vi "nanocal -- nuclear schottky fit V8.vi"() -> ()   [LabVIEW 2021] (continued)
0.011257222829   ,  \"σηlogτN\" -> 0.184131010310   ,  \"σlogτ1\" -> 0.004582504926   ,  \"σlogτS\" -> 0.002840955825   ,  \"σlogτN\" -> 0.002523601752   ,  \"σητ1\" -> 0.013755317417   ,  \"σητS \" -> 0.001255629993   ,  \"σητN\" -> 0.084667169226    |>   , \r\"IDS0627_220611_RAW_cal__sam_\" ->   <|    \"ζ\" -> 0.000000000000   ,  \"τ1\" -> 0.000000000000   ,  \"τS\" -> 0.000000000000   ,  \"τN\" -> 0.000000000000   ,  \"τC\" -> 0.000000000000   ,  \"κ0\" -> 0.000000000000   ,  \"mm1\" -> 0.000000000000   ,  \"mm2\" -> 0.000000000000   ,  \"mm3\" -> 0.000000000000   ,  \"T\" -> 0.120000000000   ,  \"B\" -> 10.000000000000   ,  \"θ\" -> 90.000000000000   ,  \"Reoff\" -> 0.000000000000   ,  \"Imoff\" -> 0.000000000000   ,  \"στ1\" -> 0.000000000000   ,  \"στS\" -> 0.000000000000   ,  \"στN\" -> 0.000000000000   ,  \"τ11 \" -> 0.000000000000   ,  \"τ12\" -> 0.000000000000   ,  \"τ22\" -> 0.000000000000   ,  \"τN1\" -> 0.000000000000   ,  \"τN2\" -> 0.000000000000   ,  \"σηlogτ1 \" -> 0.000000000000   ,  \"σηlogτS\" -> 0.000000000000   ,  \"σηlogτN\" -> 0.000000000000   ,  \"σlogτ1\" -> 0.000000000000   ,  \"σlogτS\" -> 0.000000000000   ,  \"σlogτN\" -> 0.000000000000   ,  \"σητ1\" -> 0.000000000000   ,  \"σητS \" -> 0.000000000000   ,  \"σητN\" -> 0.000000000000    |>   , \r\"IDS0628_220611_RAW_cal__ref_\" ->   <|    \"ζ\" -> 0.152770220737   ,  \"τ1\" -> 0.036198364925   ,  \"τS\" -> 0.033549808091   ,  \"τN\" -> 0.027206802922   ,  \"τC\" -> 0.001036197063   ,  \"κ0\" -> 0.000000001265   ,  \"mm1\" -> 0.000134182447   ,  \"mm2\" -> 0.015662270095   ,  \"mm3\" -> 0.091476521334   ,  \"T\" -> 0.250000000000   ,  \"B\" -> 10.000000000000   ,  \"θ\" -> 90.000000000000   ,  \"Reoff\" -> 0.000000000000   ,  \"Imoff\" -> 0.000000000000   ,  \"στ1\" -> 0.000013390131   ,  \"στS\" -> 0.000002421606   ,  \"στN\" -> 0.000006177026   ,  \"τ11 \" -> 0.000000000000   ,  \"τ12\" -> 0.000000000000   ,  \"τ22\" -> 0.000000000000   ,  \"τN1\" -> 0.000000000000   ,  \"τN2\" -> 0.000000000000   ,  \"σηlogτ1 \" -> 0.116147333813   ,  \"σηlogτS\" -> 0.002721053400   ,  \"σηlogτN\" -> 0.134955883548   ,  \"σlogτ1\" -> 0.000369909834   ,  \"σlogτS\" -> 0.000072179437   ,  \"σlogτN\" -> 0.000227039759   ,  \"σητ1\" -> 0.004204343574   ,  \"σητS \" -> 0.000091290819   ,  \"σητN\" -> 0.003671718127    |>   , \r\"IDS0628_220611_RAW_cal__sam_\" ->   <|    \"ζ\" -> 0.000000000000   ,  \"τ1\" -> 0.000000000000   ,  \"τS\" -> 0.000000000000   ,  \"τN\" -> 0.000000000000   ,  \"τC\" -> 0.000000000000   ,  \"κ0\" -> 0.000000000000   ,  \"mm1\" -> 0.000000000000   ,  \"mm2\" -> 0.000000000000   ,  \"mm3\" -> 0.000000000000   ,  \"T\" -> 0.250000000000   ,  \"B\" -> 10.000000000000   ,  \"θ\" -> 90.000000000000   ,  \"Reoff\" -> 0.000000000000   ,  \"Imoff\" -> 0.000000000000   ,  \"στ1\" -> 0.000000000000   ,  \"στS\" -> 0.000000000000   ,  \"στN\" -> 0.000000000000   ,  \"τ11 \" -> 0.000000000000   ,  \"τ12\" -> 0.000000000000   ,  \"τ22\" -> 0.000000000000   ,  \"τN1\" -> 0.000000000000   ,  \"τN2\" -> 0.000000000000   ,  \"σηlogτ1 \" -> 0.000000000000   ,  \"σηlogτS\" -> 0.000000000000   ,  \"σηlogτN\" -> 0.000000000000   ,  \"σlogτ1\" -> 0.000000000000   ,  \"σlogτS\" -> 0.000000000000   ,  \"σlogτN\" -> 0.000000000000   ,  \"σητ1\" -> 0.000000000000   ,  \"σητS \" -> 0.000000000000   ,  \"σητN\" -> 0.000000000000    |>   , \r\"IDS0629_220611_RAW_cal__ref_\" ->   <|    \"ζ\" -> 0.104961058193   ,  \"τ1\" -> 0.030489437824   ,  \"τS\" -> 0.030011872176   ,  \"τN\" -> 0.014021025099   ,  \"τC\" -> 0.001158647608   ,  \"κ0\" -> 0.000000001606   ,  \"mm1\" -> 0.000106671353   ,  \"mm2\" -> 0.016335963882   ,  \"mm3\" -> 0.063860086965   ,  \"T\" -> 0.300000000000   ,  \"B\" -> 10.000000000000   ,  \"θ\" -> 90.000000000000   ,  \"Reoff\" -> 0.000000000000   ,  \"Imoff\" -> 0.000000000000   ,  \"στ1\" -> 0.000007085631   ,  \"στS\" -> 0.000000880275   ,  \"στN\" -> 0.000001925171   ,  \"τ11 \" -> 0.000000000000   ,  \"τ12\" -> 0.000000000000   ,  \"τ22\" -> 0.000000000000   ,  \"τN1\" -> 0.000000000000   ,  \"τN2\" -> 0.000000000000   ,  \"σηlogτ1 \" -> 0.117123612292   ,  \"σηlogτS\" -> 0.001807335056   ,  \"σηlogτN\" -> 0.132991316128   ,  \"σlogτ1\" -> 0.000232396245   ,  \"σlogτS\" -> 0.000029330901   ,  \"σlogτN\" -> 0.000137306042   ,  \"σητ1\" -> 0.003571033095   ,  \"σητS \" -> 0.000054241509   ,  \"σητN\" -> 0.001864674581    |>   , \r\"IDS0629_220611_RAW_cal__sam_\" ->   <|    \"ζ\" -> 0.000000000000   ,  \"τ1\" -> 0.000000000000   ,  \"τS\" -> 0.000000000000   ,  \"τN\" -> 0.000000000000   ,  \"τC\" -> 0.000000000000   ,  \"κ0\" -> 0.000000000000   ,  \"mm1\" -> 0.000000000000   ,  \"mm2\" -> 0.000000000000   ,  \"mm3\" -> 0.000000000000   ,  \"T\" -> 0.300000000000   ,  \"B\" -> 10.000000000000   ,  \"θ\" -> 90.000000000000   ,  \"Reoff\" -> 0.000000000000   ,  \"Imoff\" -> 0.000000000000   ,  \"στ1\" -> 0.000000000000   ,  \"στS\" -> 0.000000000000   ,  \"στN\" -> 0.000000000000   ,  \"τ11 \" -> 0.000000000000   ,  \"τ12\" -> 0.000000000000   ,  \"τ22\" -> 0.000000000000   ,  \"τN1\" -> 0.000000000000   ,  \"τN2\" -> 0.000000000000   ,  \"σηlogτ1 \" -> 0.000000000000   ,  \"σηlogτS\" -> 0.000000000000   ,  \"σηlogτN\" -> 0.000000000000   ,  \"σlogτ1\" -> 0.000000000000   ,  \"σlogτS\" -> 0.000000000000   ,  \"σlogτN\" -> 0.000000000000   ,  \"σητ1\" -> 0.000000000000   ,  \"σητS \" -> 0.000000000000   ,  \"σητN\" -> 0.000000000000    |>   , \r\"IDS0630_220611_RAW_cal__ref_\" ->   <|    \"ζ\" -> 0.075687079530   ,  \"τ1\" -> 0.025692917456   ,  \"τS\" -> 0.027518005635   ,  \"τN\" -> 0.007256477389   ,  \"τC\" -> 0.001413406836   ,  \"κ0\" -> 0.000000002017   ,  \"mm1\" -> 0.000095205662   ,  \"mm2\" -> 0.016621150094   ,  \"mm3\" -> 0.047796430622   ,  \"T\" -> 0.360000000000   ,  \"B\" -> 10.000000000000   ,  \"θ\" -> 90.000000000000   ,  \"Reoff\" -> 0.000000000000   ,  \"Imoff\" -> 0.000000000000   ,  \"στ1\" -> 0.000009211361   ,  \"στS\" -> 0.000000780336   ,  \"στN\" -> 0.000001470575   ,  \"τ11 \" -> 0.000000000000   ,  \"τ12\" -> 0.000000000000   ,  \"τ22\" -> 0.000000000000   ,  \"τN1\" -> 0.000000000000   ,  \"τN2\" -> 0.000000000000   ,  \"σηlogτ1 \" -> 0.121353390675   ,  \"σηlogτS\" -> 0.001216073528   ,  \"σηlogτN\" -> 0.132703139128   ,  \"σlogτ1\" -> 0.000358517508   ,  \"σlogτS\" -> 0.000028357288   ,  \"σlogτN\" -> 0.000202656857   ,  \"σητ1\" -> 0.003117922650   ,  \"σητS \" -> 0.000033463918   ,  \"σητN\" -> 0.000962957328    |>   , \r\"IDS0630_220611_RAW_cal__sam_\" ->   <|    \"ζ\" -> 0.000000000000   ,  \"τ1\" -> 0.000000000000   ,  \"τS\" -> 0.000000000000   ,  \"τN\" -> 0.000000000000   ,  \"τC\" -> 0.000000000000   ,  \"κ0\" -> 0.000000000000   ,  \"mm1\" -> 0.000000000000   ,  \"mm2\" -> 0.000000000000   ,  \"mm3\" -> 0.000000000000   ,  \"T\" -> 0.360000000000   ,  \"B\" -> 10.000000000000   ,  \"θ\" -> 90.000000000000   ,  \"Reoff\" -> 0.000000000000   ,  \"Imoff\" -> 0.000000000000   ,  \"στ1\" -> 0.000000000000   ,  \"στS\" -> 0.000000000000   ,  \"στN\" -> 0.000000000000   ,  \"τ11 \" -> 0.000000000000   ,  \"τ12\" -> 0.000000000000   ,  \"τ22\" -> 0.000000000000   ,  \"τN1\" -> 0.000000000000   ,  \"τN2\" -> 0.000000000000   ,  \"σηlogτ1 \" -> 0.000000000000   ,  \"σηlogτS\" -> 0.000000000000   ,  \"σηlogτN\" -> 0.000000000000   ,  \"σlogτ1\" -> 0.000000000000   ,  \"σlogτS\" -> 0.000000000000   ,  \"σlogτN\" -> 0.000000000000   ,  \"σητ1\" -> 0.000000000000   ,  \"σητS \" -> 0.000000000000   ,  \"σητN\" -> 0.000000000000    |>   , \r\"IDS0631_220611_RAW_cal__ref_\" ->   <|    \"ζ\" -> 0.058935240336   ,  \"τ1\" -> 0.021193518217   ,  \"τS\" -> 0.025799898485   ,  \"τN\" -> 0.004769009758   ,  \"τC\" -> 0.001612077295   ,  \"κ0\" -> 0.000000002413   ,  \"mm1\" -> 0.000084967559   ,  \"mm2\" -> 0.015406650385   ,  \"mm3\" -> 0.039684471765   ,  \"T\" -> 0.420000000000   ,  \"B\" -> 10.000000000000   ,  \"θ\" -> 90.000000000000   ,  \"Reoff\" -> 0.000000000000   ,  \"Imoff\" -> 0.000000000000   ,  \"στ1\" -> 0.000010740234   ,  \"στS\" -> 0.000000797297   ,  \"στN\" -> 0.000001307044   ,  \"τ11 \" -> 0.000000000000   ,  \"τ12\" -> 0.000000000000   ,  \"τ22\" -> 0.000000000000   ,  \"τN1\" -> 0.000000000000   ,  \"τN2\" -> 0.000000000000   ,  \"σηlogτ1 \" -> 0.129682628231   ,  \"σηlogτS\" -> 0.001061043633   ,  \"σηlogτN\" -> 0.134054055610   ,  \"σlogτ1\" -> 0.000506769772   ,  \"σlogτS\" -> 0.000030903120   ,  \"σlogτN\" -> 0.000274070212   ,  \"σητ1\" -> 0.002748431144   ,  \"σητS \" -> 0.000027374818   ,  \"σητN\" -> 0.000639305099    |>   , \r\"IDS0631_220611_RAW_cal__sam_\" ->   <|    \"ζ\" -> 0.000000000000   ,  \"τ1\" -> 0.000000000000   ,  \"τS\" -> 0.000000000000   ,  \"τN\" -> 0.000000000000   ,  \"τC\" -> 0.000000000000   ,  \"κ0\" -> 0.000000000000   ,  \"mm1\" -> 0.000000000000   ,  \"mm2\" -> 0.000000000000   ,  \"mm3\" -> 0.000000000000   ,  \"T\" -> 0.420000000000   ,  \"B\" -> 10.000000000000   ,  \"θ\" -> 90.000000000000   ,  \"Reoff\" -> 0.000000000000   ,  \"Imoff\" -> 0.000000000000   ,  \"στ1\" -> 0.000000000000   ,  \"στS\" -> 0.000000000000   ,  \"στN\" -> 0.000000000000   ,  \"τ11 \" -> 0.000000000000   ,  \"τ12\" -> 0.000000000000   ,  \"τ22\" -> 0.000000000000   ,  \"τN1\" -> 0.000000000000   ,  \"τN2\" -> 0.000000000000   ,  \"σηlogτ1 \" -> 0.000000000000   ,  \"σηlogτS\" -> 0.000000000000   ,  \"σηlogτN\" -> 0.000000000000   ,  \"σlogτ1\" -> 0.000000000000   ,  \"σlogτS\" -> 0.000000000000   ,  \"σlogτN\" -> 0.000000000000   ,  \"σητ1\" -> 0.000000000000   ,  \"σητS \" -> 0.000000000000   ,  \"σητN\" -> 0.000000000000    |>   , \r\"IDS0632_220611_RAW_cal__ref_\" ->   <|    \"ζ\" -> 0.044055217720   ,  \"τ1\" -> 0.018398673141   ,  \"τS\" -> 0.024296902753   ,  \"τN\" -> 0.002237219247   ,  \"τC\" -> 0.001705422897   ,  \"κ0\" -> 0.000000003103   ,  \"mm1\" -> 0.000067596634   ,  \"mm2\" -> 0.015331750366   ,  \"mm3\" -> 0.032407837560   ,  \"T\" -> 0.520000000000   ,  \"B\" -> 10.000000000000   ,  \"θ\" -> 90.000000000000   ,  \"Reoff\" -> 0.000000000000   ,  \"Imoff\" -> 0.000000000000   ,  \"στ1\" -> 0.000025900073   ,  \"στS\" -> 0.000001114973   ,  \"στN\" -> 0.000001649689   ,  \"τ11 \" -> 0.000000000000   ,  \"τ12\" -> 0.000000000000   ,  \"τ22\" -> 0.000000000000   ,  \"τN1\" -> 0.000000000000   ,  \"τN2\" -> 0.000000000000   ,  \"σηlogτ1 \" -> 0.135453082912   ,  \"σηlogτS\" -> 0.000614451179   ,  \"σηlogτN\" -> 0.134477904132   ,  \"σlogτ1\" -> 0.001407714152   ,  \"σlogτS\" -> 0.000045889504   ,  \"σlogτN\" -> 0.000737383723   ,  \"σητ1\" -> 0.002492156998   ,  \"σητS \" -> 0.000014929261   ,  \"σητN\" -> 0.000300856555    |>   , \r\"IDS0632_220611_RAW_cal__sam_\" ->   <|    \"ζ\" -> 0.000000000000   ,  \"τ1\" -> 0.000000000000   ,  \"τS\" -> 0.000000000000   ,  \"τN\" -> 0.000000000000   ,  \"τC\" -> 0.000000000000   ,  \"κ0\" -> 0.000000000000   ,  \"mm1\" -> 0.000000000000   ,  \"mm2\" -> 0.000000000000   ,  \"mm3\" -> 0.000000000000   ,  \"T\" -> 0.520000000000   ,  \"B\" -> 10.000000000000   ,  \"θ\" -> 90.000000000000   ,  \"Reoff\" -> 0.000000000000   ,  \"Imoff\" -> 0.000000000000   ,  \"στ1\" -> 0.000000000000   ,  \"στS\" -> 0.000000000000   ,  \"στN\" -> 0.000000000000   ,  \"τ11 \" -> 0.000000000000   ,  \"τ12\" -> 0.000000000000   ,  \"τ22\" -> 0.000000000000   ,  \"τN1\" -> 0.000000000000   ,  \"τN2\" -> 0.000000000000   ,  \"σηlogτ1 \" -> 0.000000000000   ,  \"σηlogτS\" -> 0.000000000000   ,  \"σηlogτN\" -> 0.000000000000   ,  \"σlogτ1\" -> 0.000000000000   ,  \"σlogτS\" -> 0.000000000000   ,  \"σlogτN\" -> 0.000000000000   ,  \"σητ1\" -> 0.000000000000   ,  \"σητS \" -> 0.000000000000   ,  \"σητN\" -> 0.000000000000    |>   , \r\"IDS0633_220611_RAW_cal__ref_\" ->   <|    \"ζ\" -> 0.034142201059   ,  \"τ1\" -> 0.016889163361   ,  \"τS\" -> 0.022852529077   ,  \"τN\" -> 0.001326577994   ,  \"τC\" -> 0.002278925943   ,  \"κ0\" -> 0.000000003798   ,  \"mm1\" -> 0.000068802803   ,  \"mm2\" -> 0.014993961538   ,  \"mm3\" -> 0.029109959968   ,  \"T\" -> 0.620000000000   ,  \"B\" -> 10.000000000000   ,  \"θ\" -> 90.000000000000   ,  \"Reoff\" -> 0.000000000000   ,  \"Imoff\" -> 0.000000000000   ,  \"στ1\" -> 0.000028192933   ,  \"στS\" -> 0.000000811322   ,  \"στN\" -> 0.000001142735   ,  \"τ11 \" -> 0.000000000000   ,  \"τ12\" -> 0.000000000000   ,  \"τ22\" -> 0.000000000000   ,  \"τN1\" -> 0.000000000000   ,  \"τN2\" -> 0.000000000000   ,  \"σηlogτ1 \" -> 0.138852812126   ,  \"σηlogτS\" -> 0.000419923481   ,  \"σηlogτN\" -> 0.134804184987   ,  \"σlogτ1\" -> 0.001669291277   ,  \"σlogτS\" -> 0.000035502510   ,  \"σlogτN\" -> 0.000861415426   ,  \"σητ1\" -> 0.002345107827   ,  \"σητS \" -> 0.000009596314   ,  \"σητN\" -> 0.000178828265    |>   , \r\"IDS0633_220611_RAW_cal__sam_\" ->   <|    \"ζ\" -> 0.000000000000   ,  \"τ1\" -> 0.000000000000   ,  \"τS\" -> 0.000000000000   ,  \"τN\" -> 0.000000000000   ,  \"τC\" -> 0.000000000000   ,  \"κ0\" -> 0.000000000000   ,  \"mm1\" -> 0.000000000000   ,  \"mm2\" -> 0.000000000000   ,  \"mm3\" -> 0.000000000000   ,  \"T\" -> 0.620000000000   ,  \"B\" -> 10.000000000000   ,  \"θ\" -> 90.000000000000   ,  \"Reoff\" -> 0.000000000000   ,  \"Imoff\" -> 0.000000000000   ,  \"στ1\" -> 0.000000000000   ,  \"στS\" -> 0.000000000000   ,  \"στN\" -> 0.000000000000   ,  \"τ11 \" -> 0.000000000000   ,  \"τ12\" -> 0.000000000000   ,  \"τ22\" -> 0.000000000000   ,  \"τN1\" -> 0.000000000000   ,  \"τN2\" -> 0.000000000000   ,  \"σηlogτ1 \" -> 0.000000000000   ,  \"σηlogτS\" -> 0.000000000000   ,  \"σηlogτN\" -> 0.000000000000   ,  \"σlogτ1\" -> 0.000000000000   ,  \"σlogτS\" -> 0.000000000000   ,  \"σlogτN\" -> 0.000000000000   ,  \"σητ1\" -> 0.000000000000   ,  \"σητS \" -> 0.000000000000   ,  \"σητN\" -> 0.000000000000    |>   , \r\"IDS0634_220612_RAW_cal__ref_\" ->   <|    \"ζ\" -> 0.026094794498   ,  \"τ1\" -> 0.017613964803   ,  \"τS\" -> 0.020608194694   ,  \"τN\" -> 0.000565779347   ,  \"τC\" -> 0.002821541401   ,  \"κ0\" -> 0.000000005177   ,  \"mm1\" -> 0.000063475218   ,  \"mm2\" -> 0.016356491351   ,  \"mm3\" -> 0.025742044177   ,  \"T\" -> 0.820000000000   ,  \"B\" -> 10.000000000000   ,  \"θ\" -> 90.000000000000   ,  \"Reoff\" -> 0.000000000000   ,  \"Imoff\" -> 0.000000000000   ,  \"στ1\" -> 0.000096609701   ,  \"στS\" -> 0.000001077026   ,  \"στN\" -> 0.000001637448   ,  \"τ11 \" -> 0.000000000000   ,  \"τ12\" -> 0.000000000000   ,  \"τ22\" -> 0.000000000000   ,  \"τN1\" -> 0.000000000000   ,  \"τN2\" -> 0.000000000000   ,  \"σηlogτ1 \" -> 0.129941381525   ,  \"σηlogτS\" -> 0.000167044779   ,  \"σηlogτN\" -> 0.132803601967   ,  \"σlogτ1\" -> 0.005484835568   ,  \"σlogτS\" -> 0.000052262034   ,  \"σlogτN\" -> 0.002894146508   ,  \"σητ1\" -> 0.002288782921   ,  \"σητS \" -> 0.000003442491   ,  \"σητN\" -> 0.000075137535    |>   , \r\"IDS0634_220612_RAW_cal__sam_\" ->   <|    \"ζ\" -> 0.000000000000   ,  \"τ1\" -> 0.000000000000   ,  \"τS\" -> 0.000000000000   ,  \"τN\" -> 0.000000000000   ,  \"τC\" -> 0.000000000000   ,  \"κ0\" -> 0.000000000000   ,  \"mm1\" -> 0.000000000000   ,  \"mm2\" -> 0.000000000000   ,  \"mm3\" -> 0.000000000000   ,  \"T\" -> 0.820000000000   ,  \"B\" -> 10.000000000000   ,  \"θ\" -> 90.000000000000   ,  \"Reoff\" -> 0.000000000000   ,  \"Imoff\" -> 0.000000000000   ,  \"στ1\" -> 0.000000000000   ,  \"στS\" -> 0.000000000000   ,  \"στN\" -> 0.000000000000   ,  \"τ11 \" -> 0.000000000000   ,  \"τ12\" -> 0.000000000000   ,  \"τ22\" -> 0.000000000000   ,  \"τN1\" -> 0.000000000000   ,  \"τN2\" -> 0.000000000000   ,  \"σηlogτ1 \" -> 0.000000000000   ,  \"σηlogτS\" -> 0.000000000000   ,  \"σηlogτN\" -> 0.000000000000   ,  \"σlogτ1\" -> 0.000000000000   ,  \"σlogτS\" -> 0.000000000000   ,  \"σlogτN\" -> 0.000000000000   ,  \"σητ1\" -> 0.000000000000   ,  \"σητS \" -> 0.000000000000   ,  \"σητN\" -> 0.000000000000    |>   , \r\"IDS0635_220612_RAW_cal__ref_\" ->   <|    \"ζ\" -> 0.022302849506   ,  \"τ1\" -> 0.019271147098   ,  \"τS\" -> 0.018127459113   ,  \"τN\" -> 0.000191566174   ,  \"τC\" -> 0.003097458701   ,  \"κ0\" -> 0.000000007267   ,  \"mm1\" -> 0.000058053364   ,  \"mm2\" -> 0.018210505050   ,  \"mm3\" -> 0.022827639136   ,  \"T\" -> 1.120000000000   ,  \"B\" -> 10.000000000000   ,  \"θ\" -> 90.000000000000   ,  \"Reoff\" -> 0.000000000000   ,  \"Imoff\" -> 0.000000000000   ,  \"στ1\" -> 0.000470741477   ,  \"στS\" -> 0.000001456602   ,  \"στN\" -> 0.000002601409   ,  \"τ11 \" -> 0.000000000000   ,  \"τ12\" -> 0.000000000000   ,  \"τ22\" -> 0.000000000000   ,  \"τN1\" -> 0.000000000000   ,  \"τN2\" -> 0.000000000000   ,  \"σηlogτ1 \" -> 0.117167586135   ,  \"σηlogτS\" -> 0.000047458198   ,  \"σηlogτN\" -> 0.130090926522   ,  \"σlogτ1\" -> 0.024427268103   ,  \"σlogτS\" -> 0.000080353339   ,  \"σlogτN\" -> 0.013579690528   ,  \"σητ1\" -> 0.002257953787   ,  \"σητS \" -> 0.000000860297   ,  \"σητN\" -> 0.000024921021    |>   , \r\"IDS0635_220612_RAW_cal__sam_\" ->   <|    \"ζ\" -> 0.000000000000   ,  \"τ1\" -> 0.000000000000   ,  \"τS\" -> 0.000000000000   ,  \"τN\" -> 0.000000000000   ,  \"τC\" -> 0.000000000000   ,  \"κ0\" -> 0.000000000000   ,  \"mm1\" -> 0.000000000000   ,  \"mm2\" -> 0.000000000000   ,  \"mm3\" -> 0.000000000000   ,  \"T\" -> 1.120000000000   ,  \"B\" -> 10.000000000000   ,  \"θ\" -> 90.000000000000   ,  \"Reoff\" -> 0.000000000000   ,  \"Imoff\" -> 0.000000000000   ,  \"στ1\" -> 0.000000000000   ,  \"στS\" -> 0.000000000000   ,  \"στN\" -> 0.000000000000   ,  \"τ11 \" -> 0.000000000000   ,  \"τ12\" -> 0.000000000000   ,  \"τ22\" -> 0.000000000000   ,  \"τN1\" -> 0.000000000000   ,  \"τN2\" -> 0.000000000000   ,  \"σηlogτ1 \" -> 0.000000000000   ,  \"σηlogτS\" -> 0.000000000000   ,  \"σηlogτN\" -> 0.000000000000   ,  \"σlogτ1\" -> 0.000000000000   ,  \"σlogτS\" -> 0.000000000000   ,  \"σlogτN\" -> 0.000000000000   ,  \"σητ1\" -> 0.000000000000   ,  \"σητS \" -> 0.000000000000   ,  \"σητN\" -> 0.000000000000    |>   , \r\"IDS0636_220612_RAW_cal__ref_\" ->   <|    \"ζ\" -> 0.017149890612   ,  \"τ1\" -> 0.022569079306   ,  \"τS\" -> 0.013897839626   ,  \"τN\" -> 0.000042116682   ,  \"τC\" -> 0.002942632523   ,  \"κ0\" -> 0.000000012622   ,  \"mm1\" -> 0.000041165605   ,  \"mm2\" -> 0.016909717625   ,  \"mm3\" -> 0.022739853633   ,  \"T\" -> 1.900000000000   ,  \"B\" -> 10.000000000000   ,  \"θ\" -> 90.000000000000   ,  \"Reoff\" -> 0.000000000000   ,  \"Imoff\" -> 0.000000000000   ,  \"στ1\" -> 0.001616870383   ,  \"στS\" -> 0.000000714504   ,  \"στN\" -> 0.000001915578   ,  \"τ11 \" -> 0.000000000000   ,  \"τ12\" -> 0.000000000000   ,  \"τ22\" -> 0.000000000000   ,  \"τN1\" -> 0.000000000000   ,  \"τN2\" -> 0.000000000000   ,  \"σηlogτ1 \" -> 0.096802089984   ,  \"σηlogτS\" -> 0.000006983072   ,  \"σηlogτN\" -> 0.125439998859   ,  \"σlogτ1\" -> 0.071640954450   ,  \"σlogτS\" -> 0.000051411167   ,  \"σlogτN\" -> 0.045482634513   ,  \"σητ1\" -> 0.002184734046   ,  \"σητS \" -> 0.000000097050   ,  \"σητN\" -> 0.000005283117    |>   , \r\"IDS0636_220612_RAW_cal__sam_\" ->   <|    \"ζ\" -> 0.000000000000   ,  \"τ1\" -> 0.000000000000   ,  \"τS\" -> 0.000000000000   ,  \"τN\" -> 0.000000000000   ,  \"τC\" -> 0.000000000000   ,  \"κ0\" -> 0.000000000000   ,  \"mm1\" -> 0.000000000000   ,  \"mm2\" -> 0.000000000000   ,  \"mm3\" -> 0.000000000000   ,  \"T\" -> 1.900000000000   ,  \"B\" -> 10.000000000000   ,  \"θ\" -> 90.000000000000   ,  \"Reoff\" -> 0.000000000000   ,  \"Imoff\" -> 0.000000000000   ,  \"στ1\" -> 0.000000000000   ,  \"στS\" -> 0.000000000000   ,  \"στN\" -> 0.000000000000   ,  \"τ11 \" -> 0.000000000000   ,  \"τ12\" -> 0.000000000000   ,  \"τ22\" -> 0.000000000000   ,  \"τN1\" -> 0.000000000000   ,  \"τN2\" -> 0.000000000000   ,  \"σηlogτ1 \" -> 0.000000000000   ,  \"σηlogτS\" -> 0.000000000000   ,  \"σηlogτN\" -> 0.000000000000   ,  \"σlogτ1\" -> 0.000000000000   ,  \"σlogτS\" -> 0.000000000000   ,  \"σlogτN\" -> 0.000000000000   ,  \"σητ1\" -> 0.000000000000   ,  \"σητS \" -> 0.000000000000   ,  \"σητN\" -> 0.000000000000    |>   , \r\"IDS0637_220612_RAW_cal__ref_\" ->   <|    \"ζ\" -> 0.017770105668   ,  \"τ1\" -> 0.021549186615   ,  \"τS\" -> 0.009965620739   ,  \"τN\" -> 0.000008203122   ,  \"τC\" -> 0.002636418134   ,  \"κ0\" -> 0.000000022540   ,  \"mm1\" -> 0.000036639898   ,  \"mm2\" -> 0.012730445827   ,  \"mm3\" -> 0.021569578789   ,  \"T\" -> 3.100000000000   ,  \"B\" -> 10.000000000000   ,  \"θ\" -> 90.000000000000   ,  \"Reoff\" -> -204081.632653061300   ,  \"Imoff\" -> 0.000000000000   ,  \"στ1\" -> 0.714525927996   ,  \"στS\" -> 0.000197909015   ,  \"στN\" -> 0.366603423191   ,  \"τ11 \" -> 0.000000000000   ,  \"τ12\" -> 0.000000000000   ,  \"τ22\" -> 0.000000000000   ,  \"τN1\" -> 0.000000000000   ,  \"τN2\" -> 0.000000000000   ,  \"σηlogτ1 \" -> 0.000000000000   ,  \"σηlogτS\" -> 0.000000000000   ,  \"σηlogτN\" -> 0.000000000000   ,  \"σlogτ1\" -> 0.000000000000   ,  \"σlogτS\" -> 0.000000000000   ,  \"σlogτN\" -> 0.000000000000   ,  \"σητ1\" -> 0.000000000000   ,  \"σητS \" -> 0.000000000000   ,  \"σητN\" -> 0.000000000000    |>   , \r\"IDS0637_220612_RAW_cal__sam_\" ->   <|    \"ζ\" -> 0.000000000000   ,  \"τ1\" -> 0.000000000000   ,  \"τS\" -> 0.000000000000   ,  \"τN\" -> 0.000000000000   ,  \"τC\" -> 0.000000000000   ,  \"κ0\" -> 0.000000000000   ,  \"mm1\" -> 0.000000000000   ,  \"mm2\" -> 0.000000000000   ,  \"mm3\" -> 0.000000000000   ,  \"T\" -> 3.100000000000   ,  \"B\" -> 10.000000000000   ,  \"θ\" -> 90.000000000000   ,  \"Reoff\" -> 0.000000000000   ,  \"Imoff\" -> 0.000000000000   ,  \"στ1\" -> 0.000000000000   ,  \"στS\" -> 0.000000000000   ,  \"στN\" -> 0.000000000000   ,  \"τ11 \" -> 0.000000000000   ,  \"τ12\" -> 0.000000000000   ,  \"τ22\" -> 0.000000000000   ,  \"τN1\" -> 0.000000000000   ,  \"τN2\" -> 0.000000000000   ,  \"σηlogτ1 \" -> 0.000000000000   ,  \"σηlogτS\" -> 0.000000000000   ,  \"σηlogτN\" -> 0.000000000000   ,  \"σlogτ1\" -> 0.000000000000   ,  \"σlogτS\" -> 0.000000000000   ,  \"σlogτN\" -> 0.000000000000   ,  \"σητ1\" -> 0.000000000000   ,  \"σητS \" -> 0.000000000000   ,  \"σητN\" -> 0.000000000000    |>   , \r\"IDS0638_220612_RAW_cal__ref_\" ->   <|    \"ζ\" -> 0.021698598791   ,  \"τ1\" -> 0.021496688345   ,  \"τS\" -> 0.006445256992   ,  \"τN\" -> 0.000001238561   ,  \"τC\" -> 0.001823286983   ,  \"κ0\" -> 0.000000055353   ,  \"mm1\" -> 0.000030436072   ,  \"mm2\" -> 0.008377153736   ,  \"mm3\" -> 0.021498760993   ,  \"T\" -> 5.700000000000   ,  \"B\" -> 10.000000000000   ,  \"θ\" -> 90.000000000000   ,  \"Reoff\" -> -122448.979591835290   ,  \"Imoff\" -> 0.000000000000   ,  \"στ1\" -> 9.353728365028   ,  \"στS\" -> 0.000421905194   ,  \"στN\" -> 5.932285308296   ,  \"τ11 \" -> 0.000000000000   ,  \"τ12\" -> 0.000000000000   ,  \"τ22\" -> 0.000000000000   ,  \"τN1\" -> 0.000000000000   ,  \"τN2\" -> 0.000000000000   ,  \"σηlogτ1 \" -> 0.000000000000   ,  \"σηlogτS\" -> 0.000000000000   ,  \"σηlogτN\" -> 0.000000000000   ,  \"σlogτ1\" -> 0.000000000000   ,  \"σlogτS\" -> 0.000000000000   ,  \"σlogτN\" -> 0.000000000000   ,  \"σητ1\" -> 0.000000000000   ,  \"σητS \" -> 0.000000000000   ,  \"σητN\" -> 0.000000000000    |>   , \r\"IDS0638_220612_RAW_cal__sam_\" ->   <|    \"ζ\" -> 0.000000000000   ,  \"τ1\" -> 0.000000000000   ,  \"τS\" -> 0.000000000000   ,  \"τN\" -> 0.000000000000   ,  \"τC\" -> 0.000000000000   ,  \"κ0\" -> 0.000000000000   ,  \"mm1\" -> 0.000000000000   ,  \"mm2\" -> 0.000000000000   ,  \"mm3\" -> 0.000000000000   ,  \"T\" -> 5.700000000000   ,  \"B\" -> 10.000000000000   ,  \"θ\" -> 90.000000000000   ,  \"Reoff\" -> 0.000000000000   ,  \"Imoff\" -> 0.000000000000   ,  \"στ1\" -> 0.000000000000   ,  \"στS\" -> 0.000000000000   ,  \"στN\" -> 0.000000000000   ,  \"τ11 \" -> 0.000000000000   ,  \"τ12\" -> 0.000000000000   ,  \"τ22\" -> 0.000000000000   ,  \"τN1\" -> 0.000000000000   ,  \"τN2\" -> 0.000000000000   ,  \"σηlogτ1 \" -> 0.000000000000   ,  \"σηlogτS\" -> 0.000000000000   ,  \"σηlogτN\" -> 0.000000000000   ,  \"σlogτ1\" -> 0.000000000000   ,  \"σlogτS\" -> 0.000000000000   ,  \"σlogτN\" -> 0.000000000000   ,  \"σητ1\" -> 0.000000000000   ,  \"σητS \" -> 0.000000000000   ,  \"σητN\" -> 0.000000000000    |>   , \r\"IDS0640_220612_RAW_cal__ref_\" ->   <|    \"ζ\" -> 0.230099904219   ,  \"τ1\" -> 0.019803524287   ,  \"τS\" -> 0.072771074412   ,  \"τN\" -> 0.019721178899   ,  \"τC\" -> 0.000908013791   ,  \"κ0\" -> 0.000000000947   ,  \"mm1\" -> 0.000168456164   ,  \"mm2\" -> 0.014977374492   ,  \"mm3\" -> 0.119340419361   ,  \"T\" -> 0.200000000000   ,  \"B\" -> 6.000000000000   ,  \"θ\" -> 90.000000000000   ,  \"Reoff\" -> 0.000000000000   ,  \"Imoff\" -> 0.000000000000   ,  \"στ1\" -> 0.000071902729   ,  \"στS\" -> 0.000035418419   ,  \"στN\" -> 0.000036759818   ,  \"τ11 \" -> 0.000000000000   ,  \"τ12\" -> 0.000000000000   ,  \"τ22\" -> 0.000000000000   ,  \"τN1\" -> 0.000000000000   ,  \"τN2\" -> 0.000000000000   ,  \"σηlogτ1 \" -> 0.251384540647   ,  \"σηlogτS\" -> 0.006630640632   ,  \"σηlogτN\" -> 0.159565745714   ,  \"σlogτ1\" -> 0.003630804676   ,  \"σlogτS\" -> 0.000486710132   ,  \"σlogτN\" -> 0.001863976680   ,  \"σητ1\" -> 0.004978299856   ,  \"σητS \" -> 0.000482518843   ,  \"σητN\" -> 0.003146824617    |>   , \r\"IDS0640_220612_RAW_cal__sam_\" ->   <|    \"ζ\" -> 0.000000000000   ,  \"τ1\" -> 0.000000000000   ,  \"τS\" -> 0.000000000000   ,  \"τN\" -> 0.000000000000   ,  \"τC\" -> 0.000000000000   ,  \"κ0\" -> 0.000000000000   ,  \"mm1\" -> 0.000000000000   ,  \"mm2\" -> 0.000000000000   ,  \"mm3\" -> 0.000000000000   ,  \"T\" -> 0.200000000000   ,  \"B\" -> 6.000000000000   ,  \"θ\" -> 90.000000000000   ,  \"Reoff\" -> 0.000000000000   ,  \"Imoff\" -> 0.000000000000   ,  \"στ1\" -> 0.000000000000   ,  \"στS\" -> 0.000000000000   ,  \"στN\" -> 0.000000000000   ,  \"τ11 \" -> 0.000000000000   ,  \"τ12\" -> 0.000000000000   ,  \"τ22\" -> 0.000000000000   ,  \"τN1\" -> 0.000000000000   ,  \"τN2\" -> 0.000000000000   ,  \"σηlogτ1 \" -> 0.000000000000   ,  \"σηlogτS\" -> 0.000000000000   ,  \"σηlogτN\" -> 0.000000000000   ,  \"σlogτ1\" -> 0.000000000000   ,  \"σlogτS\" -> 0.000000000000   ,  \"σlogτN\" -> 0.000000000000   ,  \"σητ1\" -> 0.000000000000   ,  \"σητS \" -> 0.000000000000   ,  \"σητN\" -> 0.000000000000    |>   , \r\"IDS0641_220612_RAW_cal__ref_\" ->   <|    \"ζ\" -> 0.331411916516   ,  \"τ1\" -> 0.027436942180   ,  \"τS\" -> 0.091259190003   ,  \"τN\" -> 0.036352249292   ,  \"τC\" -> 0.000814813533   ,  \"κ0\" -> 0.000000000745   ,  \"mm1\" -> 0.000201800322   ,  \"mm2\" -> 0.018690769514   ,  \"mm3\" -> 0.179262576839   ,  \"T\" -> 0.170000000000   ,  \"B\" -> 6.000000000000   ,  \"θ\" -> 90.000000000000   ,  \"Reoff\" -> 0.000000000000   ,  \"Imoff\" -> 0.000000000000   ,  \"στ1\" -> 0.000134182156   ,  \"στS\" -> 0.000082842638   ,  \"στN\" -> 0.000089641447   ,  \"τ11 \" -> 0.000000000000   ,  \"τ12\" -> 0.000000000000   ,  \"τ22\" -> 0.000000000000   ,  \"τN1\" -> 0.000000000000   ,  \"τN2\" -> 0.000000000000   ,  \"σηlogτ1 \" -> 0.243050215213   ,  \"σηlogτS\" -> 0.008562643138   ,  \"σηlogτN\" -> 0.162803839532   ,  \"σlogτ1\" -> 0.004890565241   ,  \"σlogτS\" -> 0.000907773107   ,  \"σlogτN\" -> 0.002465911967   ,  \"σητ1\" -> 0.006668554702   ,  \"σητS \" -> 0.000781419877   ,  \"σητN\" -> 0.005918285760    |>   , \r\"IDS0641_220612_RAW_cal__sam_\" ->   <|    \"ζ\" -> 0.000000000000   ,  \"τ1\" -> 0.000000000000   ,  \"τS\" -> 0.000000000000   ,  \"τN\" -> 0.000000000000   ,  \"τC\" -> 0.000000000000   ,  \"κ0\" -> 0.000000000000   ,  \"mm1\" -> 0.000000000000   ,  \"mm2\" -> 0.000000000000   ,  \"mm3\" -> 0.000000000000   ,  \"T\" -> 0.170000000000   ,  \"B\" -> 6.000000000000   ,  \"θ\" -> 90.000000000000   ,  \"Reoff\" -> 0.000000000000   ,  \"Imoff\" -> 0.000000000000   ,  \"στ1\" -> 0.000000000000   ,  \"στS\" -> 0.000000000000   ,  \"στN\" -> 0.000000000000   ,  \"τ11 \" -> 0.000000000000   ,  \"τ12\" -> 0.000000000000   ,  \"τ22\" -> 0.000000000000   ,  \"τN1\" -> 0.000000000000   ,  \"τN2\" -> 0.000000000000   ,  \"σηlogτ1 \" -> 0.000000000000   ,  \"σηlogτS\" -> 0.000000000000   ,  \"σηlogτN\" -> 0.000000000000   ,  \"σlogτ1\" -> 0.000000000000   ,  \"σlogτS\" -> 0.000000000000   ,  \"σlogτN\" -> 0.000000000000   ,  \"σητ1\" -> 0.000000000000   ,  \"σητS \" -> 0.000000000000   ,  \"σητN\" -> 0.000000000000    |>   , \r\"IDS0642_220612_RAW_cal__ref_\" ->   <|    \"ζ\" -> 0.410773621242   ,  \"τ1\" -> 0.031455114933   ,  \"τS\" -> 0.109824084123   ,  \"τN\" -> 0.054894161716   ,  \"τC\" -> 0.000807067579   ,  \"κ0\" -> 0.000000000644   ,  \"mm1\" -> 0.000234124076   ,  \"mm2\" -> 0.020015527109   ,  \"mm3\" -> 0.244392687495   ,  \"T\" -> 0.150000000000   ,  \"B\" -> 6.000000000000   ,  \"θ\" -> 90.000000000000   ,  \"Reoff\" -> 0.000000000000   ,  \"Imoff\" -> 0.000000000000   ,  \"στ1\" -> 0.000244365389   ,  \"στS\" -> 0.000194798011   ,  \"στN\" -> 0.000213345438   ,  \"τ11 \" -> 0.000000000000   ,  \"τ12\" -> 0.000000000000   ,  \"τ22\" -> 0.000000000000   ,  \"τN1\" -> 0.000000000000   ,  \"τN2\" -> 0.000000000000   ,  \"σηlogτ1 \" -> 0.251218681926   ,  \"σηlogτS\" -> 0.010865743955   ,  \"σηlogτN\" -> 0.168296468755   ,  \"σlogτ1\" -> 0.007768701196   ,  \"σlogτS\" -> 0.001773727614   ,  \"σlogτN\" -> 0.003886486855   ,  \"σητ1\" -> 0.007902112513   ,  \"σητS \" -> 0.001193320378   ,  \"σητN\" -> 0.009238493572    |>   , \r\"IDS0642_220612_RAW_cal__sam_\" ->   <|    \"ζ\" -> 0.000000000000   ,  \"τ1\" -> 0.000000000000   ,  \"τS\" -> 0.000000000000   ,  \"τN\" -> 0.000000000000   ,  \"τC\" -> 0.000000000000   ,  \"κ0\" -> 0.000000000000   ,  \"mm1\" -> 0.000000000000   ,  \"mm2\" -> 0.000000000000   ,  \"mm3\" -> 0.000000000000   ,  \"T\" -> 0.150000000000   ,  \"B\" -> 6.000000000000   ,  \"θ\" -> 90.000000000000   ,  \"Reoff\" -> 0.000000000000   ,  \"Imoff\" -> 0.000000000000   ,  \"στ1\" -> 0.000000000000   ,  \"στS\" -> 0.000000000000   ,  \"στN\" -> 0.000000000000   ,  \"τ11 \" -> 0.000000000000   ,  \"τ12\" -> 0.000000000000   ,  \"τ22\" -> 0.000000000000   ,  \"τN1\" -> 0.000000000000   ,  \"τN2\" -> 0.000000000000   ,  \"σηlogτ1 \" -> 0.000000000000   ,  \"σηlogτS\" -> 0.000000000000   ,  \"σηlogτN\" -> 0.000000000000   ,  \"σlogτ1\" -> 0.000000000000   ,  \"σlogτS\" -> 0.000000000000   ,  \"σlogτN\" -> 0.000000000000   ,  \"σητ1\" -> 0.000000000000   ,  \"σητS \" -> 0.000000000000   ,  \"σητN\" -> 0.000000000000    |>   , \r\"IDS0643_220612_RAW_cal__ref_\" ->   <|    \"ζ\" -> 0.645665826507   ,  \"τ1\" -> 0.033591555956   ,  \"τS\" -> 0.115598019979   ,  \"τN\" -> 0.189817561833   ,  \"τC\" -> 0.000794602780   ,  \"κ0\" -> 0.000000000472   ,  \"mm1\" -> 0.000310954135   ,  \"mm2\" -> 0.012215752320   ,  \"mm3\" -> 0.524471438152   ,  \"T\" -> 0.120000000000   ,  \"B\" -> 6.000000000000   ,  \"θ\" -> 90.000000000000   ,  \"Reoff\" -> -174187755.102040827000   ,  \"Imoff\" -> 0.000000000000   ,  \"στ1\" -> 0.039640874529   ,  \"στS\" -> 0.065981071320   ,  \"στN\" -> 0.095740947662   ,  \"τ11 \" -> 0.000000000000   ,  \"τ12\" -> 0.000000000000   ,  \"τ22\" -> 0.000000000000   ,  \"τN1\" -> 0.000000000000   ,  \"τN2\" -> 0.000000000000   ,  \"σηlogτ1 \" -> 0.000000000000   ,  \"σηlogτS\" -> 0.000000000000   ,  \"σηlogτN\" -> 0.000000000000   ,  \"σlogτ1\" -> 0.000000000000   ,  \"σlogτS\" -> 0.000000000000   ,  \"σlogτN\" -> 0.000000000000   ,  \"σητ1\" -> 0.000000000000   ,  \"σητS \" -> 0.000000000000   ,  \"σητN\" -> 0.000000000000    |>   , \r\"IDS0643_220612_RAW_cal__sam_\" ->   <|    \"ζ\" -> 0.000000000000   ,  \"τ1\" -> 0.000000000000   ,  \"τS\" -> 0.000000000000   ,  \"τN\" -> 0.000000000000   ,  \"τC\" -> 0.000000000000   ,  \"κ0\" -> 0.000000000000   ,  \"mm1\" -> 0.000000000000   ,  \"mm2\" -> 0.000000000000   ,  \"mm3\" -> 0.000000000000   ,  \"T\" -> 0.120000000000   ,  \"B\" -> 6.000000000000   ,  \"θ\" -> 90.000000000000   ,  \"Reoff\" -> 0.000000000000   ,  \"Imoff\" -> 0.000000000000   ,  \"στ1\" -> 0.000000000000   ,  \"στS\" -> 0.000000000000   ,  \"στN\" -> 0.000000000000   ,  \"τ11 \" -> 0.000000000000   ,  \"τ12\" -> 0.000000000000   ,  \"τ22\" -> 0.000000000000   ,  \"τN1\" -> 0.000000000000   ,  \"τN2\" -> 0.000000000000   ,  \"σηlogτ1 \" -> 0.000000000000   ,  \"σηlogτS\" -> 0.000000000000   ,  \"σηlogτN\" -> 0.000000000000   ,  \"σlogτ1\" -> 0.000000000000   ,  \"σlogτS\" -> 0.000000000000   ,  \"σlogτN\" -> 0.000000000000   ,  \"σητ1\" -> 0.000000000000   ,  \"σητS \" -> 0.000000000000   ,  \"σητN\" -> 0.000000000000    |>   , \r\"IDS0644_220612_RAW_cal__ref_\" ->   <|    \"ζ\" -> 0.157159831769   ,  \"τ1\" -> 0.017275661419   ,  \"τS\" -> 0.057507819747   ,  \"τN\" -> 0.009018768853   ,  \"τC\" -> 0.000968005523   ,  \"κ0\" -> 0.000000001253   ,  \"mm1\" -> 0.000129832569   ,  \"mm2\" -> 0.014431696620   ,  \"mm3\" -> 0.080664033826   ,  \"T\" -> 0.250000000000   ,  \"B\" -> 6.000000000000   ,  \"θ\" -> 90.000000000000   ,  \"Reoff\" -> 0.000000000000   ,  \"Imoff\" -> 0.000000000000   ,  \"στ1\" -> 0.000090637790   ,  \"στS\" -> 0.000023650584   ,  \"στN\" -> 0.000024208134   ,  \"τ11 \" -> 0.000000000000   ,  \"τ12\" -> 0.000000000000   ,  \"τ22\" -> 0.000000000000   ,  \"τN1\" -> 0.000000000000   ,  \"τN2\" -> 0.000000000000   ,  \"σηlogτ1 \" -> 0.236297448492   ,  \"σηlogτS\" -> 0.003600470511   ,  \"σηlogτN\" -> 0.153004528887   ,  \"σlogτ1\" -> 0.005246559741   ,  \"σlogτS\" -> 0.000411258583   ,  \"σlogτN\" -> 0.002684194999   ,  \"σητ1\" -> 0.004082194714   ,  \"σητS \" -> 0.000207055209   ,  \"σητN\" -> 0.001379912479    |>   , \r\"IDS0644_220612_RAW_cal__sam_\" ->   <|    \"ζ\" -> 0.000000000000   ,  \"τ1\" -> 0.000000000000   ,  \"τS\" -> 0.000000000000   ,  \"τN\" -> 0.000000000000   ,  \"τC\" -> 0.000000000000   ,  \"κ0\" -> 0.000000000000   ,  \"mm1\" -> 0.000000000000   ,  \"mm2\" -> 0.000000000000   ,  \"mm3\" -> 0.000000000000   ,  \"T\" -> 0.250000000000   ,  \"B\" -> 6.000000000000   ,  \"θ\" -> 90.000000000000   ,  \"Reoff\" -> 0.000000000000   ,  \"Imoff\" -> 0.000000000000   ,  \"στ1\" -> 0.000000000000   ,  \"στS\" -> 0.000000000000   ,  \"στN\" -> 0.000000000000   ,  \"τ11 \" -> 0.000000000000   ,  \"τ12\" -> 0.000000000000   ,  \"τ22\" -> 0.000000000000   ,  \"τN1\" -> 0.000000000000   ,  \"τN2\" -> 0.000000000000   ,  \"σηlogτ1 \" -> 0.000000000000   ,  \"σηlogτS\" -> 0.000000000000   ,  \"σηlogτN\" -> 0.000000000000   ,  \"σlogτ1\" -> 0.000000000000   ,  \"σlogτS\" -> 0.000000000000   ,  \"σlogτN\" -> 0.000000000000   ,  \"σητ1\" -> 0.000000000000   ,  \"σητS \" -> 0.000000000000   ,  \"σητN\" -> 0.000000000000    |>   , \r\"IDS0645_220612_RAW_cal__ref_\" ->   <|    \"ζ\" -> 0.108151444543   ,  \"τ1\" -> 0.016704569544   ,  \"τS\" -> 0.049250197086   ,  \"τN\" -> 0.004328811909   ,  \"τC\" -> 0.001175701627   ,  \"κ0\" -> 0.000000001596   ,  \"mm1\" -> 0.000112550307   ,  \"mm2\" -> 0.014943415376   ,  \"mm3\" -> 0.062197961703   ,  \"T\" -> 0.300000000000   ,  \"B\" -> 6.000000000000   ,  \"θ\" -> 90.000000000000   ,  \"Reoff\" -> 0.000000000000   ,  \"Imoff\" -> 0.000000000000   ,  \"στ1\" -> 0.000153951281   ,  \"στS\" -> 0.000019651803   ,  \"στN\" -> 0.000020146314   ,  \"τ11 \" -> 0.000000000000   ,  \"τ12\" -> 0.000000000000   ,  \"τ22\" -> 0.000000000000   ,  \"τN1\" -> 0.000000000000   ,  \"τN2\" -> 0.000000000000   ,  \"σηlogτ1 \" -> 0.218575565601   ,  \"σηlogτS\" -> 0.001786286514   ,  \"σηlogτN\" -> 0.148268126955   ,  \"σlogτ1\" -> 0.009216117846   ,  \"σlogτS\" -> 0.000399019782   ,  \"σlogτN\" -> 0.004654005435   ,  \"σητ1\" -> 0.003651210736   ,  \"σητS \" -> 0.000087974963   ,  \"σητN\" -> 0.000641824834    |>   , \r\"IDS0645_220612_RAW_cal__sam_\" ->   <|    \"ζ\" -> 0.000000000000   ,  \"τ1\" -> 0.000000000000   ,  \"τS\" -> 0.000000000000   ,  \"τN\" -> 0.000000000000   ,  \"τC\" -> 0.000000000000   ,  \"κ0\" -> 0.000000000000   ,  \"mm1\" -> 0.000000000000   ,  \"mm2\" -> 0.000000000000   ,  \"mm3\" -> 0.000000000000   ,  \"T\" -> 0.300000000000   ,  \"B\" -> 6.000000000000   ,  \"θ\" -> 90.000000000000   ,  \"Reoff\" -> 0.000000000000   ,  \"Imoff\" -> 0.000000000000   ,  \"στ1\" -> 0.000000000000   ,  \"στS\" -> 0.000000000000   ,  \"στN\" -> 0.000000000000   ,  \"τ11 \" -> 0.000000000000   ,  \"τ12\" -> 0.000000000000   ,  \"τ22\" -> 0.000000000000   ,  \"τN1\" -> 0.000000000000   ,  \"τN2\" -> 0.000000000000   ,  \"σηlogτ1 \" -> 0.000000000000   ,  \"σηlogτS\" -> 0.000000000000   ,  \"σηlogτN\" -> 0.000000000000   ,  \"σlogτ1\" -> 0.000000000000   ,  \"σlogτS\" -> 0.000000000000   ,  \"σlogτN\" -> 0.000000000000   ,  \"σητ1\" -> 0.000000000000   ,  \"σητS \" -> 0.000000000000   ,  \"σητN\" -> 0.000000000000    |>   , \r\"IDS0646_220612_RAW_cal__ref_\" ->   <|    \"ζ\" -> 0.077732977787   ,  \"τ1\" -> 0.018222452777   ,  \"τS\" -> 0.042664974364   ,  \"τN\" -> 0.002414957753   ,  \"τC\" -> 0.001447490324   ,  \"κ0\" -> 0.000000001997   ,  \"mm1\" -> 0.000101431981   ,  \"mm2\" -> 0.016791513450   ,  \"mm3\" -> 0.051361127148   ,  \"T\" -> 0.360000000000   ,  \"B\" -> 6.000000000000   ,  \"θ\" -> 90.000000000000   ,  \"Reoff\" -> 0.000000000000   ,  \"Imoff\" -> 0.000000000000   ,  \"στ1\" -> 0.000164595012   ,  \"στS\" -> 0.000010037791   ,  \"στN\" -> 0.000010800479   ,  \"τ11 \" -> 0.000000000000   ,  \"τ12\" -> 0.000000000000   ,  \"τ22\" -> 0.000000000000   ,  \"τN1\" -> 0.000000000000   ,  \"τN2\" -> 0.000000000000   ,  \"σηlogτ1 \" -> 0.189495281548   ,  \"σηlogτS\" -> 0.000864174070   ,  \"σηlogτN\" -> 0.143351503659   ,  \"σlogτ1\" -> 0.009032538816   ,  \"σlogτS\" -> 0.000235270067   ,  \"σlogτN\" -> 0.004472326314   ,  \"σητ1\" -> 0.003453068820   ,  \"σητS \" -> 0.000036869965   ,  \"σητN\" -> 0.000346187825    |>   , \r\"IDS0646_220612_RAW_cal__sam_\" ->   <|    \"ζ\" -> 0.000000000000   ,  \"τ1\" -> 0.000000000000   ,  \"τS\" -> 0.000000000000   ,  \"τN\" -> 0.000000000000   ,  \"τC\" -> 0.000000000000   ,  \"κ0\" -> 0.000000000000   ,  \"mm1\" -> 0.000000000000   ,  \"mm2\" -> 0.000000000000   ,  \"mm3\" -> 0.000000000000   ,  \"T\" -> 0.360000000000   ,  \"B\" -> 6.000000000000   ,  \"θ\" -> 90.000000000000   ,  \"Reoff\" -> 0.000000000000   ,  \"Imoff\" -> 0.000000000000   ,  \"στ1\" -> 0.000000000000   ,  \"στS\" -> 0.000000000000   ,  \"στN\" -> 0.000000000000   ,  \"τ11 \" -> 0.000000000000   ,  \"τ12\" -> 0.000000000000   ,  \"τ22\" -> 0.000000000000   ,  \"τN1\" -> 0.000000000000   ,  \"τN2\" -> 0.000000000000   ,  \"σηlogτ1 \" -> 0.000000000000   ,  \"σηlogτS\" -> 0.000000000000   ,  \"σηlogτN\" -> 0.000000000000   ,  \"σlogτ1\" -> 0.000000000000   ,  \"σlogτS\" -> 0.000000000000   ,  \"σlogτN\" -> 0.000000000000   ,  \"σητ1\" -> 0.000000000000   ,  \"σητS \" -> 0.000000000000   ,  \"σητN\" -> 0.000000000000    |>   , \r\"IDS0647_220612_RAW_cal__ref_\" ->   <|    \"ζ\" -> 0.059413527113   ,  \"τ1\" -> 0.016818995328   ,  \"τS\" -> 0.037585637610   ,  \"τN\" -> 0.001580842075   ,  \"τC\" -> 0.001700025734   ,  \"κ0\" -> 0.000000002392   ,  \"mm1\" -> 0.000091637686   ,  \"mm2\" -> 0.015787959467   ,  \"mm3\" -> 0.044132922297   ,  \"T\" -> 0.420000000000   ,  \"B\" -> 6.000000000000   ,  \"θ\" -> 90.000000000000   ,  \"Reoff\" -> 0.000000000000   ,  \"Imoff\" -> 0.000000000000   ,  \"στ1\" -> 0.000108112505   ,  \"στS\" -> 0.000004614270   ,  \"στN\" -> 0.000005017637   ,  \"τ11 \" -> 0.000000000000   ,  \"τ12\" -> 0.000000000000   ,  \"τ22\" -> 0.000000000000   ,  \"τN1\" -> 0.000000000000   ,  \"τN2\" -> 0.000000000000   ,  \"σηlogτ1 \" -> 0.183880264698   ,  \"σηlogτS\" -> 0.000605017197   ,  \"σηlogτN\" -> 0.142205307504   ,  \"σlogτ1\" -> 0.006428000169   ,  \"σlogτS\" -> 0.000122766832   ,  \"σlogτN\" -> 0.003174028004   ,  \"σητ1\" -> 0.003092681313   ,  \"σητS \" -> 0.000022739957   ,  \"σητN\" -> 0.000224804133    |>   , \r\"IDS0647_220612_RAW_cal__sam_\" ->   <|    \"ζ\" -> 0.000000000000   ,  \"τ1\" -> 0.000000000000   ,  \"τS\" -> 0.000000000000   ,  \"τN\" -> 0.000000000000   ,  \"τC\" -> 0.000000000000   ,  \"κ0\" -> 0.000000000000   ,  \"mm1\" -> 0.000000000000   ,  \"mm2\" -> 0.000000000000   ,  \"mm3\" -> 0.000000000000   ,  \"T\" -> 0.420000000000   ,  \"B\" -> 6.000000000000   ,  \"θ\" -> 90.000000000000   ,  \"Reoff\" -> 0.000000000000   ,  \"Imoff\" -> 0.000000000000   ,  \"στ1\" -> 0.000000000000   ,  \"στS\" -> 0.000000000000   ,  
